vi "testTwoClientsSendTelemetryAtSameTime.vi"(8 "error in":errorcluster) -> (0 "error out":errorcluster)   [LabVIEW 2018]
uses:
  src/FactoryTcpServer/FactoryTcpServer.lvclass
  <vilib>/addons/_JKI Toolkits/Caraya/classes/Assert/Assert Equal Value_Variant.vi
  src/TcpServer/TcpServer.lvclass
  <vilib>/addons/_JKI Toolkits/Caraya/classes/Test/Test.lvclass
  <vilib>/addons/_JKI Toolkits/Caraya/classes/Assert/Assert.lvclass
panel:
  out "Run Server B error":errorcluster
  out "Run Server A error":errorcluster
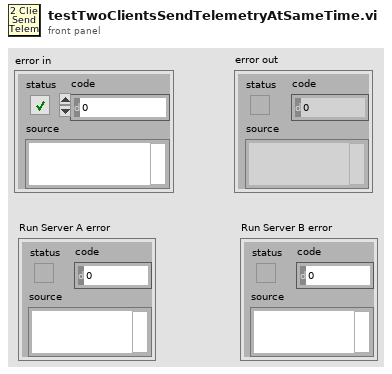
[diagram p1: front panel]
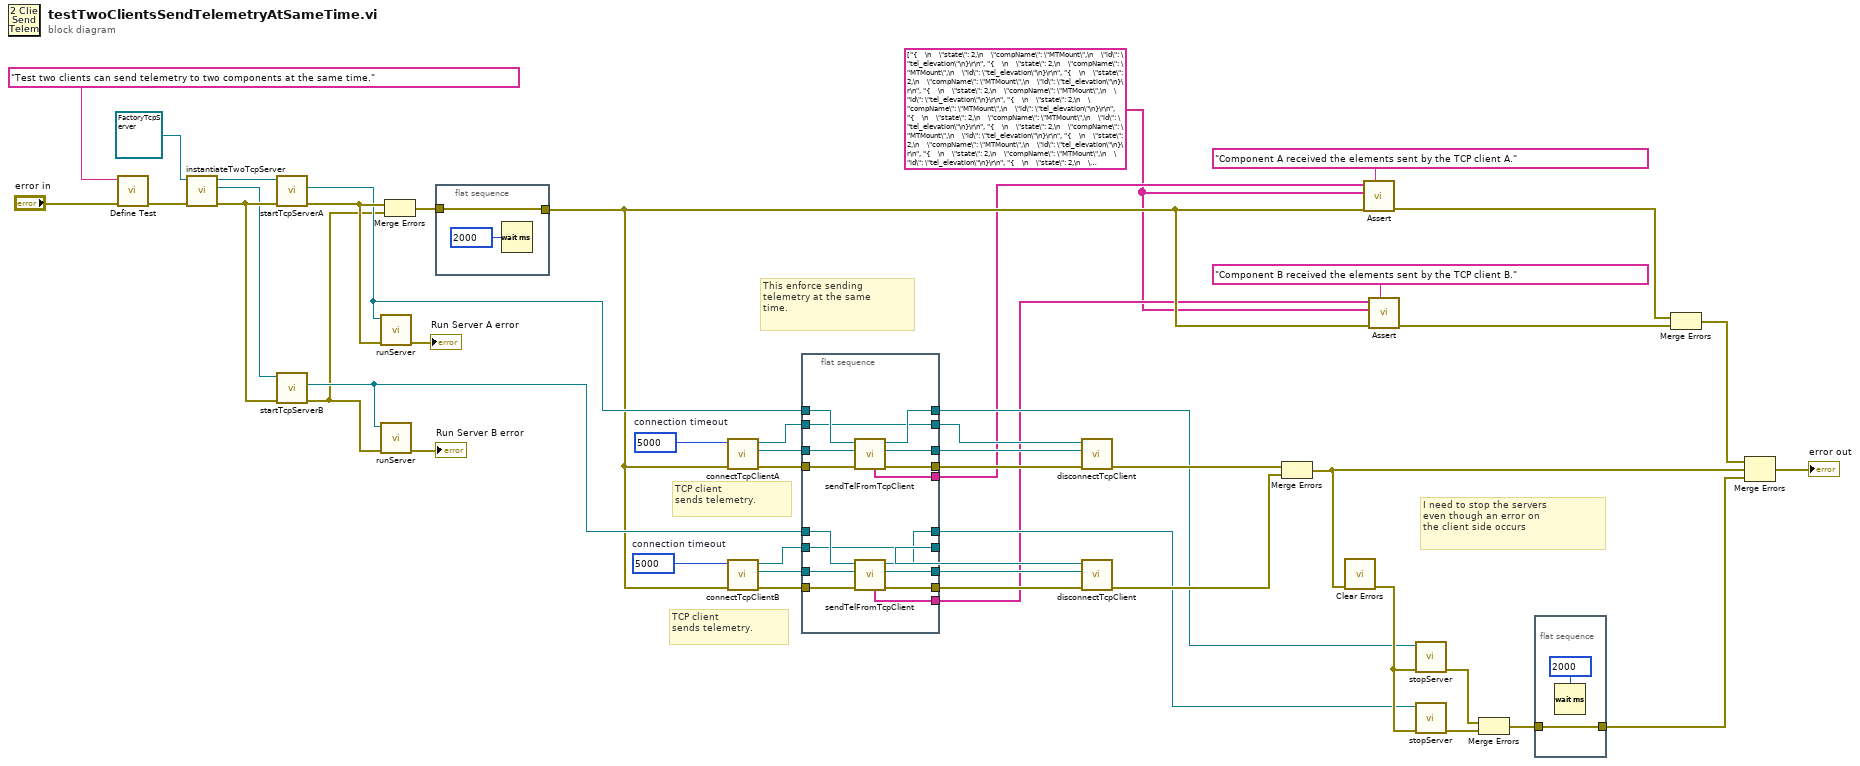
[diagram p0: block diagram]
diagram:
  w1 = string[] ["{    \n    \"state\": 2,\n    \"compName\": \"MTMount\",\n    \"id\": \"tel_elevation\"\n}\r\n", "{    \n    \"state\": 2,\n    \"compName\": \"MTMount\",\n    \"id\": \"tel_elevation\"\n}\r\n", "{    \n    \"state\": 2,\n    \"compName\": \"MTMount\",\n    \"id\": \"tel_elevation\"\n}\r\n", "{    \n    \"state\": 2,\n    \"compName\": \"MTMount\",\n    \"id\": \"tel_elevation\"\n}\r\n", "{    \n    \"state\": 2,\n    \"compName\": \"MTMount\",\n    \"id\": \"tel_elevation\"\n}\r\n", "{    \n    \"state\": 2,\n    \"compName\": \"MTMount\",\n    \"id\": \"tel_elevation\"\n}\r\n", "{    \n    \"state\": 2,\n    \"compName\": \"MTMount\",\n    \"id\": \"tel_elevation\"\n}\r\n", "{    \n    \"state\": 2,\n    \"compName\": \"MTMount\",\n    \"id\": \"tel_elevation\"\n}\r\n", "{    \n    \"state\": 2,\n    \"compName\": \"MTMount\",\n    \"id\": \"tel_elevation\"\n}\r\n", "{    \n    \"state\": 2,\n    \"compName\": \"MTMount\",\n    \"id\": \"tel_elevation\"\n}\r\n"] ("initialized array 2")
  w12 = 5000  # connection timeout
  w13 = 5000  # connection timeout
  # "TCP client \nsends telemetry."
  # "TCP client \nsends telemetry."
  # "I need to stop the servers \neven though an error on \nthe client side occurs"
  # "This enforce sending\ntelemetry at the same\ntime."
  n1 = call <vilib>:"Define Test.vi"("error in (no error)"="error in", "Label (VI Title)"="Test two clients can send telemetry to two components at the same time.") -> ("error out"=w39:errorcluster)  [unwired: 9 in]
  n2 = call "instantiateTwoTcpServer.vi"("error in (no error)"=w39, "FactoryTcpServer in"=refnum<class "FactoryTcpServer.lvclass"> refnum) -> ("error out"=w11:errorcluster, "TcpServer 2 out"=w8:refnum<class "TcpServer.lvclass">, "TcpServer 1 out"=w9:refnum<class "TcpServer.lvclass">)  [unwired: 6 in, 1 out]
  n3 = call "startTcpServerA.vi"("error in (no error)"=w11, "TcpServer.lvclass"=w9) -> ("error out"=w34:errorcluster, "TcpServer out"=w33:refnum<class "TcpServer.lvclass">)  [unwired: 7 in, 1 out]
  n4 = call "startTcpServerB.vi"("error in (no error)"=w11, "TcpServer.lvclass"=w8) -> ("error out"=w14:errorcluster, "TcpServer out"=w30:refnum<class "TcpServer.lvclass">)  [unwired: 7 in, 1 out]
  n5 = call "runServer.vi"("error in (no error)"=w34, "TcpServer in"=w33) -> ("error out (no error)"=→"Run Server A error":errorcluster)  [unwired: 8 in, 1 out]
  n6 = call "runServer.vi"("error in (no error)"=w14, "TcpServer in"=w30) -> ("error out (no error)"=→"Run Server B error":errorcluster)  [unwired: 8 in, 1 out]
  n7 = Merge Errors(w34, w14) -> (w15:errorcluster)
  n8 = flat-sequence {
    tunnel: [w49] -> w4
    tunnel: w15 -> [w49]
    frame #0 {
      n9 = Wait (ms)(milliseconds to wait=u32 2000) -> ()  [unwired: 1 out]
    }
  }
  n10 = call "connectTcpClientA.vi"("error in (no error)"=w4, "connection timeout (ms)"=w13) -> ("error out"=w7:errorcluster, "tel connection ID A out"=w24:refnum<k5>, "cmd connection ID A out"=w20:refnum<k5>)  [unwired: 7 in]
  n11 = call "connectTcpClientB.vi"("error in (no error)"=w4, "connection timeout (ms)"=w12) -> ("error out"=w26:errorcluster, "tel connection ID B out"=w28:refnum<k5>, "cmd connection ID B out"=w18:refnum<k5>)  [unwired: 7 in]
  n12 = flat-sequence {
    tunnel: w33 -> [w66]
    tunnel: [w65] -> w32
    tunnel: [w64] -> w31
    tunnel: w30 -> [w63]
    tunnel: [w52] -> w3
    tunnel: w28 -> [w62]
    tunnel: [w61] -> w27
    tunnel: w26 -> [w60]
    tunnel: [w59] -> w25
    tunnel: w24 -> [w58]
    tunnel: [w57] -> w23
    tunnel: w7 -> [w56]
    tunnel: [w55] -> w22
    tunnel: [w54] -> w21
    tunnel: w20 -> [w54]
    tunnel: [w53] -> w19
    tunnel: w18 -> [w53]
    tunnel: [w51] -> w2
    frame #0 {
      n13 = call "sendTelFromTcpClient.vi"("error in (no error)"=w56, "tel connection ID in"=w58, "TcpServer in"=w66) -> ("error out"=w55:errorcluster, "tel connection ID out"=w57:refnum<k5>, "TcpServer out"=w65:refnum<class "TcpServer.lvclass">, "telemetry received"=w52:string[])  [unwired: 4 in, 1 out]
      n14 = call "sendTelFromTcpClient.vi"("error in (no error)"=w60, "tel connection ID in"=w62, "TcpServer in"=w63) -> ("error out"=w59:errorcluster, "tel connection ID out"=w61:refnum<k5>, "TcpServer out"=w64:refnum<class "TcpServer.lvclass">, "telemetry received"=w51:string[])  [unwired: 4 in, 1 out]
    }
  }
  n15 = call "disconnectTcpClient.vi"("error in (no error)"=w22, "tel connection ID in"=w23, "cmd connection ID in"=w21) -> ("error out"=w41:errorcluster)  [unwired: 8 in]
  n16 = call "disconnectTcpClient.vi"("error in (no error)"=w25, "tel connection ID in"=w27, "cmd connection ID in"=w19) -> ("error out"=w38:errorcluster)  [unwired: 8 in]
  n17 = Merge Errors(w41, w38) -> (w36:errorcluster)
  n18 = call <vilib>:"Clear Errors.vi"("error in (no error)"=w36) -> ("error out"=w35:errorcluster)  [unwired: 5 in, 1 out]
  n19 = call-poly <vilib>:"Assert.vi"("Label"="Component A received the elements sent by the TCP client A.", "error in (no error)"=w4, "Y"=w1, "X"=w3) -> ("error out"=w17:errorcluster)  [unwired: 7 in]
  n20 = call-poly <vilib>:"Assert.vi"("Label"="Component B received the elements sent by the TCP client B.", "error in (no error)"=w4, "Y"=w1, "X"=w2) -> ("error out"=w5:errorcluster)  [unwired: 7 in]
  n21 = call "stopServer.vi"("error in (no error)"=w35, "tcpServer in"=w32) -> ("error out"=w45:errorcluster)  [unwired: 8 in, 1 out]
  n22 = call "stopServer.vi"("error in (no error)"=w35, "tcpServer in"=w31) -> ("error out"=w44:errorcluster)  [unwired: 8 in, 1 out]
  n23 = Merge Errors(w45, w44) -> (w43:errorcluster)
  n24 = flat-sequence {
    tunnel: w43 -> [w67]
    tunnel: [w67] -> w37
    frame #0 {
      n25 = Wait (ms)(milliseconds to wait=u32 2000) -> ()  [unwired: 1 out]
    }
  }
  n26 = Merge Errors(w17, w5) -> (w16:errorcluster)
  n27 = Merge Errors(w16, w36, w37) -> (→"error out":errorcluster)
